vi "RunScript.vi"(8 "ErrorArray":errorcluster[](array[cluster]), 10 "Script":string[](array[string]), 11 "Bus":refnum<class "Bus.lvclass">) -> (0 "ErrorArray":errorcluster[](array[cluster]), 2 "Data out":variant, 3 "Bus":refnum<class "Bus.lvclass">)   [LabVIEW 2014, in "Bus_class.lvlib" / "Bus.lvclass"]
uses:
  Bus.lvclass
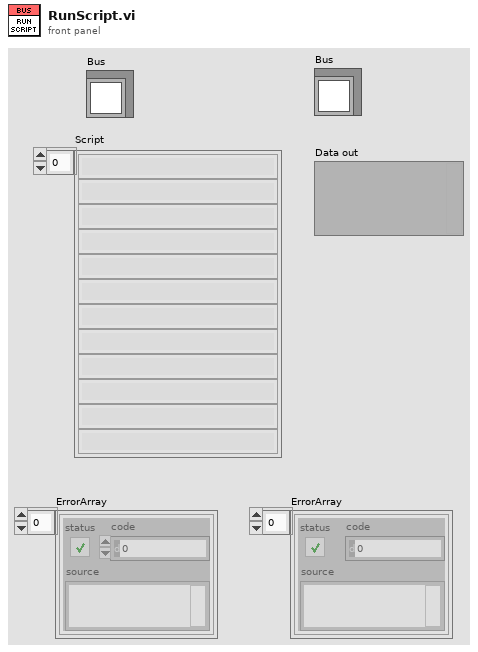
[diagram p1: front panel]
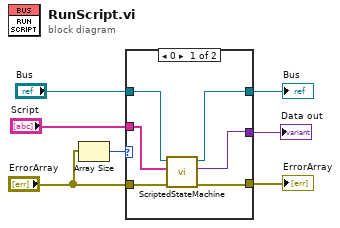
[diagram p0: block diagram]
diagram:
  n1 = Array Size(array="ErrorArray") -> (size(s)=w7:i32)
  n2 = case shown="0" w7 {
    tunnel: [w9 w15] -> w5
    tunnel: "ErrorArray" -> [w13 w15]
    tunnel: "Bus" -> [w11 w14]
    tunnel: [w10 w14] -> w3
    tunnel: "Script" -> [w12 _]
    tunnel: [w8 _] -> w1
    frame 0 {
      n3 = call "ScriptedStateMachine.vi"("ErrorArray In"=w13, "Script"=w12, "Bus"=w11) -> ("ErrorArray Out"=w9:errorcluster[], "Data out"=w8:variant, "Bus"=w10:refnum<class "Bus.lvclass">)  [unwired: 6 in]
    }
    frame 1, Default {
    }
  }
  "ErrorArray" <- w5
  "Bus" <- w3
  "Data out" <- w1
